vi "DigitalDebouncer_Example.vi"() -> ()   [LabVIEW 2019]
uses:
  <vilib>/Rock Robotics/WPI/ThirdParty/JAS_Junk/TrajLib/Enum/DEBOUNCER_TYPE_ENUM.ctl
  <vilib>/Rock Robotics/WPI/ThirdParty/JAS_Junk/TrajLib/TypeDef/DEBOUNCER.ctl
  <vilib>/Rock Robotics/WPI/ThirdParty/JAS_Junk/TrajLib/Trajectory_Library.lvlib
  <vilib>/ptbypt/NI_PtbyPt.lvlib
panel:
  in  "Bounce Len (Ms)":i32=6
  out "Input":bool
  out "Waveform Chart":cluster{i16, i16}(graph)
  in  "Input Frequency (Hz)":dbl=0.5
  out "Output":bool
  out "Debouncer":T1 {"PrevTimeSeconds" format="%13.6p"; "DebounceTimeSeconds" format="%13.6p"}
  in  "DebounceType":T2=enum."Both"
  in  "DebounceTime (Sec)":dbl=0.03
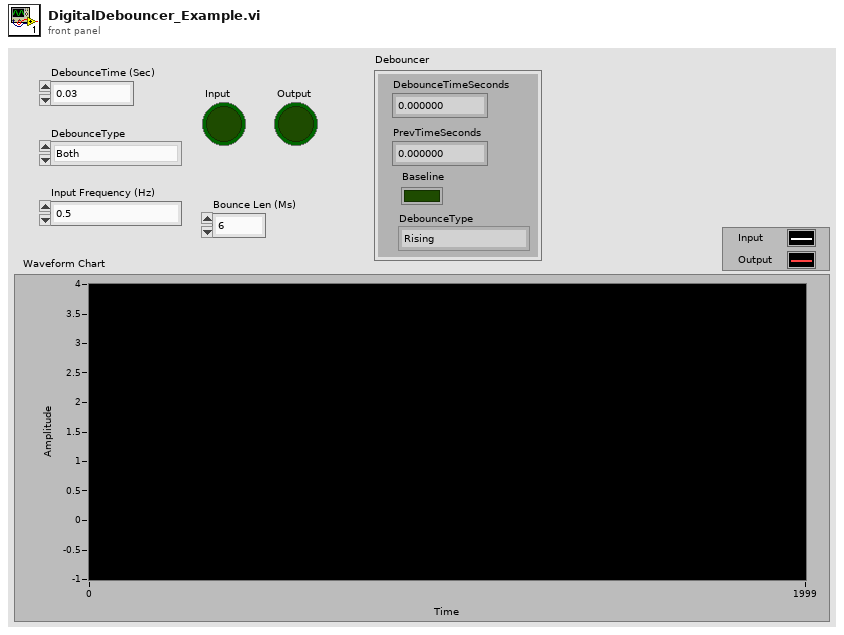
[diagram p1: front panel]
types:
  T1 = typedef "Trajectory_Library.lvlib/DEBOUNCER.ctl" = cluster{"DebounceTimeSeconds":dbl, "PrevTimeSeconds":dbl, "Baseline":bool, "DebounceType":T2}
  T2 = typedef "Trajectory_Library.lvlib/DEBOUNCER_TYPE_ENUM.ctl" = enum16{"Rising", "Falling", "Both"}
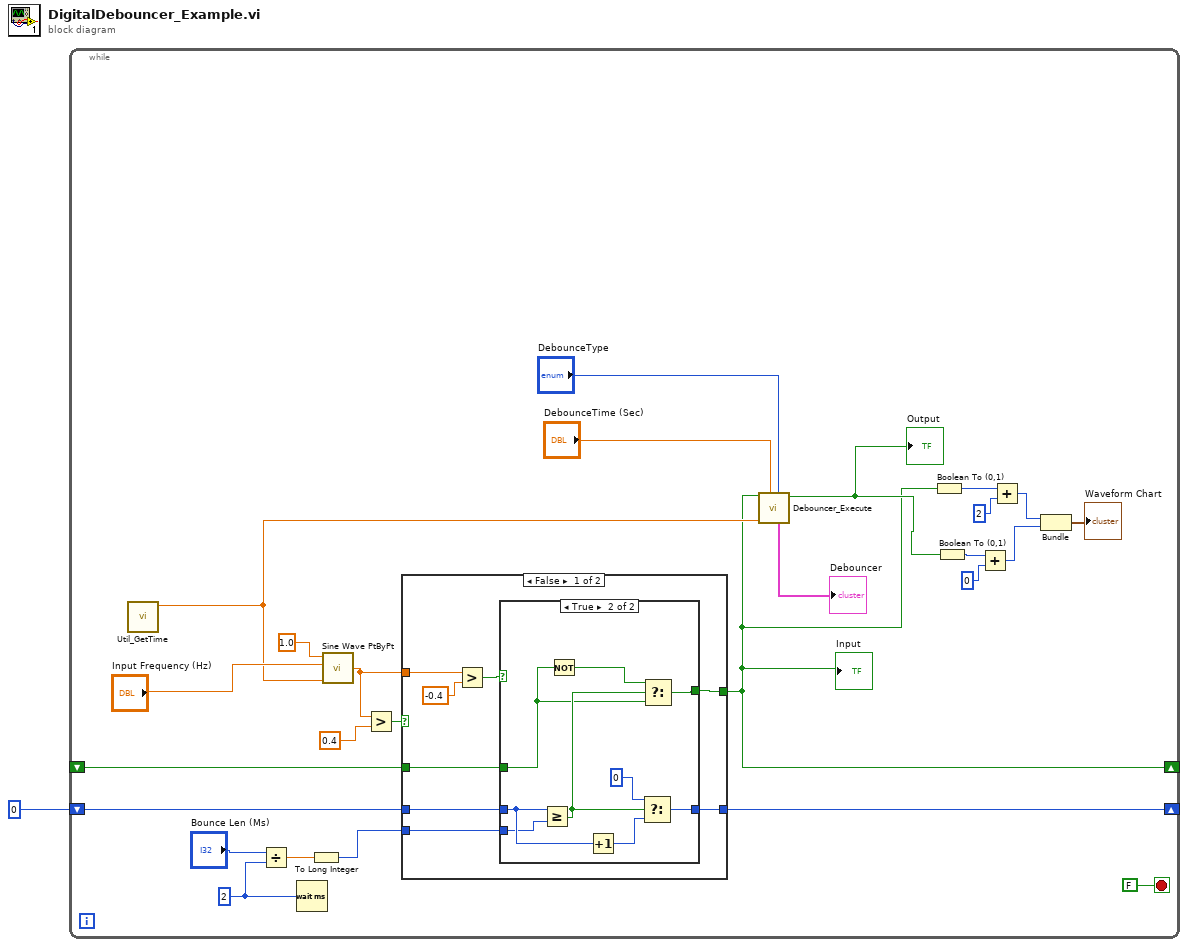
[diagram p0: block diagram]
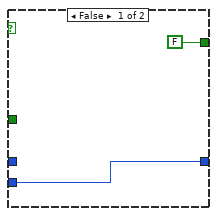
[diagram p2: hidden frame]
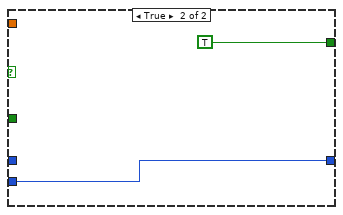
[diagram p3: hidden frame]
diagram:
  n1 = while {
    shift-right: [w7] -> _
    shift-left: 0 -> [w9]
    shift-right: [w8] -> _
    shift-left: _ -> [w6]
    stop <- FALSE stop-if-true
    w4 = u32 2 ("milliseconds to wait")
    n2 = call <vilib>:"Util_GetTime.vi"() -> ("FPGA_Time_Seconds"=w21:dbl)  [unwired: 10 in, 1 out]
    n3 = Divide(x="Bounce Len (Ms)", y=w4) -> (x/y=w2:dbl)
    n4 = Wait (ms)(milliseconds to wait=w4) -> ()  [unwired: 1 out]
    n5 = To Long Integer(number=w2) -> (32bit integer=w3:i32)
    n6 = call <vilib>:"Sine Wave PtByPt.vi"("time"=w21, "frequency"="Input Frequency (Hz)", "amplitude"=1.0) -> ("sine wave"=w10:dbl)  [unwired: 1 in]
    n7 = Greater?(x=w10, y=0.4) -> (0:w12:bool)
    n8 = case shown="False" w12 {
      tunnel: [w32 TRUE] -> w8
      tunnel: w10 -> [w35 _]
      tunnel: w9 -> [w31 _]
      tunnel: [w30 w47] -> w7
      tunnel: w6 -> [w29 _]
      tunnel: w3 -> [w28 w47]
      frame False {
        n9 = Greater?(x=w35, y=-0.4) -> (0:w33:bool)
        n10 = case shown="True" w33 {
          tunnel: [FALSE w39] -> w32
          tunnel: w31 -> [_ w45]
          tunnel: [w36 w43] -> w30
          tunnel: w29 -> [_ w41]
          tunnel: w28 -> [w36 w38]
          frame False {
          }
          frame True {
            n11 = Greater Or Equal?(x=w45, y=w38) -> (x >= y?=w42:bool)
            n12 = Not(x=w41) -> (.not. x?=w40:bool)
            n13 = Increment(x=w45) -> (x+1=w44:i32)
            n14 = Select(t=0 ("y"), s=w42, f=w44) -> (s? t:f=w43:i32)
            n15 = Select(t=w40, s=w42, f=w41) -> (s? t:f=w39:bool)
          }
        }
      }
      frame True {
      }
    }
    "Input" <- w8
    n16 = call <vilib>:"Debouncer_Execute.vi"("DebounceType"="DebounceType", "DebounceTime"="DebounceTime (Sec)", "CurrentTIme"=w21, "Input"=w8) -> ("Output"=w20:bool, "Debouncer"=→"Debouncer":T1)  [unwired: 6 in]
    "Output" <- w20
    n17 = Boolean To (0,1)(Boolean=w8) -> (0, 1=w15:i16)
    n18 = Boolean To (0,1)(Boolean=w20) -> (0, 1=w19:i16)
    n19 = Add(x=w19, y=i16 0) -> (x+y=w18:i16)
    n20 = Add(x=w15, y=i16 2) -> (x+y=w14:i16)
    n21 = Bundle(w14, w18) -> (→"Waveform Chart":cluster{i16, i16})  [unwired: 1 in]
  }
